vi "PH_BackreflectionMeas.PC Get data.vi"(0 "i ref in":refnum<vi>, 5 "error IO":errorcluster) -> (14 "i ref out":refnum<vi>, 19 "error out":errorcluster)   [LabVIEW 2014, in "PH_BackreflectionMeas.lvlib"]
doc: "This is the proc case \"Get Data\": It communicates with hardware to get data and writes them to own attributes."
uses:
  PH_BackreflectionMeas.lvlib
  PH_Devices/PH_TKTDS-30xx/PH_TKTDS-30xx.Waveform to fetch.ctl
  PH_Basics/PH_StatusHandler/PH_StatusHandler.Status.ctl
  PH_Devices/PH_TKTDS-30xx/PH_TKTDS-30xx.lvlib
  PH_Basics/PH_StatusHandler/PH_StatusHandler.lvlib
panel:
  in  "Waveform to fetch":T1={"Source"="CH1", "Waveform Start"=1, "Waveform End"=10000}
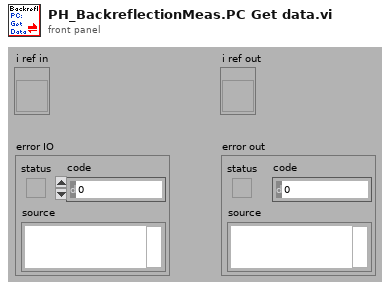
[diagram p1: front panel]
types:
  T1 = typedef "PH_TKTDS-30xx.lvlib/PH_TKTDS-30xx.Waveform to fetch.ctl" = cluster{"Source":string, "Waveform Start":i32, "Waveform End":i32}
  T2 = typedef "PH_StatusHandler.lvlib/PH_StatusHandler.Status.ctl" = i16
  T3 = typedef "PH_TKTDS-30xx.lvlib/PH_TKTDS-30xx.i attribute.ctl" = cluster{"Default VISA Resource":string, "VISA Resource Name":refnum<visa-resource-name>, "Revision":cluster{"Instrument Driver":string, "Instrument Firmware":string}, "Selftest":cluster{"Result":u32, "Message":string}, "Channels":T4[], "Trigger Configuration":T5, "Acquisition Configuration":T6, "Fetched Waveforms":T7[], "GUI Refs":T8, "GUI Refs Channels":refnum<vi>[], "State":T2, "Error Message":string, "Allow Prdc Loop?":bool}
  T4 = typedef "PH_TKTDS-30xx.lvlib/PH_TKTDS-30xx.Channel Config.ctl" = cluster{"Channel Name":string, "Input Impedance":string, "Max Input Frequency":string, "Vertical Coupling":i32, "Channel Enabled":bool, "Probe Attenuation":dbl, "Vertical Range":dbl, "Vertical Offset":dbl}
  T5 = typedef "PH_TKTDS-30xx.lvlib/PH_TKTDS-30xx.Trigger Config.ctl" = cluster{"Source":string, "Slope":i32, "Level [V]":dbl}
  T6 = typedef "PH_TKTDS-30xx.lvlib/PH_TKTDS-30xx.Acquisition Config.ctl" = cluster{"Time base":dbl, "Record Length":u16, "Start Time":dbl, "Type":i32, "Continuous":bool}
  T7 = typedef "PH_TKTDS-30xx.lvlib/PH_TKTDS-30xx.fetched Waveform.ctl" = cluster{"Source":string, "Actual Points":u32, "Initial X":dbl, "X Increment":dbl, "Waveform Array":dbl[]}
  T8 = typedef "PH_TKTDS-30xx.lvlib/PH_TKTDS-30xx.GUI Refs.ctl" = cluster{"Trigger":refnum<vi>, "Acquisition":refnum<vi>, "Graph":refnum<vi>, "State":refnum<vi>, "Delete":refnum<vi>, "Channel to be positioned":refnum<vi>, "Postion":refnum<vi>, "Display Intensity":refnum<vi>, "VISA Resource":refnum<vi>}
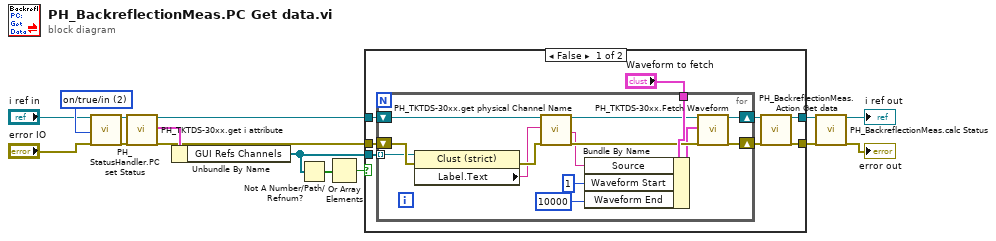
[diagram p0: block diagram]
diagram:
  w15 = T2 2 items=["no info", "off/false/out", "on/true/in", "Failure", "Alarm", "Status 1", "Status 2", "Status 3"] ("Status")
  n1 = call "PH_StatusHandler.PC set Status.vi"("i ref in"="i ref in", "Status"=w15, "error in (no error)"="error IO") -> ("i ref out"=w7:refnum<vi>, "error out"=w5:errorcluster)  [unwired: 15 in]
  n2 = call "PH_TKTDS-30xx.get i attribute.vi"("i ref in"=w7, "error in (no error)"=w5) -> ("i ref out"=w6:refnum<vi>, "i attribute"=w8:T3, "error out"=w4:errorcluster)  [unwired: 15 in]
  n3 = Unbundle By Name(w8) -> ("GUI Refs Channels"=w2:refnum<vi>[])
  n4 = Not A Number/Path/Refnum?(number/path/refnum=w2) -> (NaN/Path/Refnum?=w3:bool[])
  n5 = Or Array Elements(Boolean array=w3) -> (logical OR=w1:bool)
  n6 = case shown="False" w1 {
    tunnel: [w20 w39] -> w14
    tunnel: [w19 w38] -> w12
    tunnel: w2 -> [w18 _]
    tunnel: w6 -> [w17 w39]
    tunnel: w4 -> [w16 w38]
    frame False {
      n7 = for {
        shift-right: [w34] -> w21
        shift-left: w16 -> [w33]
        shift-right: [w35] -> w22
        shift-left: w17 -> [w36]
        tunnel: "Waveform to fetch" -> [w37]
        tunnel: w18 -> [w31] mode=indexing
        n8 = property class="Clust (strict)"(reference=w31, error in=w33) -> (error out=w32:errorcluster, "Label.Text"=w30:string)  [unwired: 1 out]
        n9 = call "PH_TKTDS-30xx.get physical Channel Name.vi"("i ref in"=w36, "GUI Element Name"=w30, "error in"=w32) -> ("i ref out"=w26:refnum<vi>, "Physical Channel Name"=w24:string, "error out"=w27:errorcluster)  [unwired: 14 in]
        n10 = Bundle By Name(cluster=w37, "Source"=w24, "Waveform Start"=1, "Waveform End"=10000) -> (w25:T1)
        n11 = call "PH_TKTDS-30xx.Fetch Waveform.vi"("i ref in"=w26, "Waveform to fetch"=w25, "error IO"=w27) -> ("i ref out"=w35:refnum<vi>, "error out"=w34:errorcluster)  [unwired: 15 in]
      }
      n12 = call "PH_BackreflectionMeas.Action Get data.vi"("i ref in"=w22, "error IO"=w21) -> ("i ref out"=w20:refnum<vi>, "error out"=w19:errorcluster)  [unwired: 16 in]
    }
    frame True {
    }
  }
  n13 = call "PH_BackreflectionMeas.calc Status.vi"("i ref in"=w14, "error in"=w12) -> ("i ref out"=→"i ref out":refnum<vi>, "error out"=→"error out":errorcluster)  [unwired: 16 in]
